vi "save_parameters_table.vi"(8 "error in":errorcluster, 10 "Parameters":T1(array[cluster]), 11 "base path":path) -> (0 "error out":errorcluster)   [LabVIEW 2012]
panel:
  out "output array":string[](array[string])
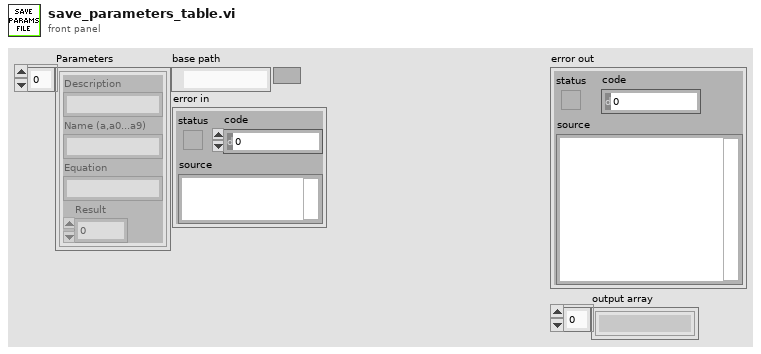
[diagram p1: front panel]
types:
  T1 = cluster{"Description":string, "Name (a,a0...a9)":string, "Equation":string, "Result":dbl}[]
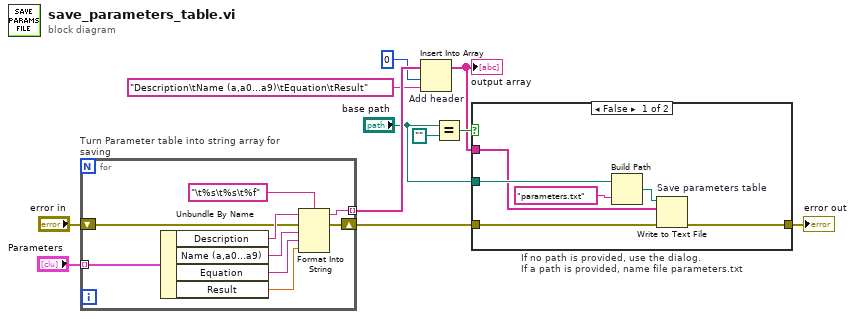
[diagram p0: block diagram]
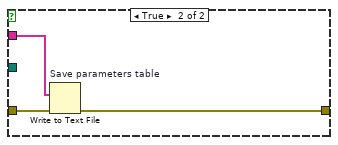
[diagram p2: hidden frame]
diagram:
  n1 = for "Turn Parameter table into string array for saving" {
    tunnel: "Parameters" -> [w20] mode=indexing
    shift-right: [w13] -> w3
    shift-left: "error in" -> [w14]
    tunnel: [w12] -> w9 mode=indexing
    n2 = Unbundle By Name(w20) -> ("Description"=w18:string, "Name (a,a0...a9)"=w17:string, "Equation"=w16:string, "Result"=w15:dbl)
    n3 = Format Into String(format string="\t%s\t%s\t%f", initial string=w18, error in=w14, w17, w16, w15) -> (resulting string=w12:string, error out=w13:errorcluster)
  }
  n4 = Insert Into Array "Add header"(array=w9, index=0, new element="Description\tName (a,a0...a9)\tEquation\tResult" ("new element/subarray")) -> (w2:string[])
  "output array" <- w2
  n5 = Equal?(x="base path", y=path "") -> (x = y?=w4:bool)
  n6 = case "If no path is provided, use the dialog.\nIf a path is provided, name file parameters.txt" shown="False" w4 {
    tunnel: [w22 w29] -> w5
    tunnel: w3 -> [w23 w28]
    tunnel: w2 -> [w21 w27]
    tunnel: "base path" -> [w25 _]
    frame False {
      n7 = Build Path(base path=w25, name or relative path="parameters.txt") -> (appended path=w24:path)
      n8 = Write to Text File "Save parameters table"(file (use dialog)=w24, text=w21, error in=w23) -> (error out=w22:errorcluster)  [unwired: 1 in, 2 out]
    }
    frame True {
      n9 = Write to Text File "Save parameters table"(text=w27, error in=w28) -> (error out=w29:errorcluster)  [unwired: 2 in, 2 out]
    }
  }
  "error out" <- w5
